vi "Logger Table.vi"() -> ()   [LabVIEW 2019]
uses:
  <vilib>/Analysis/NI_AALBase.lvlib
panel:
  out "x/y 3":dbl
  out "x/y 2":dbl
  out "x/y":dbl
  in  "Weighting (Sample)":enum16{"Sample", "Population"}(ring)
  out "standard deviation 3":dbl format="%.3f"
  out "variance 3":dbl format="%.10f"
  out "Waveform Graph":dbl[](graph)
  out "variance 2":dbl format="%.10f"
  out "variance":dbl format="%.10f"
  in  "samples":i32=100000
  out "standard deviation 2":dbl format="%.3f"
  out "standard deviation":dbl format="%.3f"
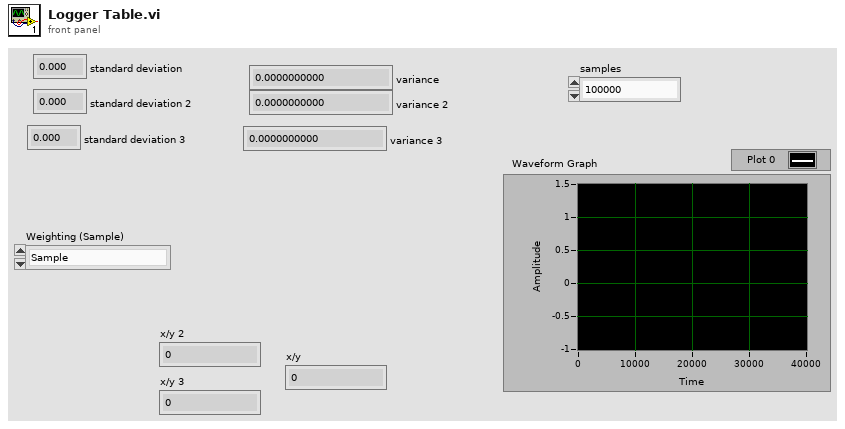
[diagram p1: front panel]
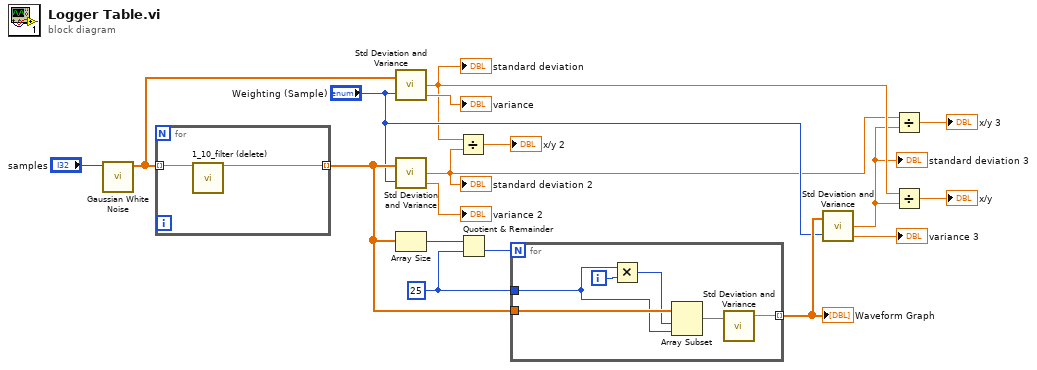
[diagram p0: block diagram]
diagram:
  w11 = 25 ("length")
  n1 = call <vilib>:"Gaussian White Noise.vi"("samples"="samples") -> ("Gaussian noise pattern"=w16:dbl[])  [unwired: 9 in, 1 out]
  n2 = for {
    tunnel: w16 -> [w18] mode=indexing
    tunnel: [w19] -> w13 mode=indexing
    n3 = call "1_10_filter (delete).vi"("input"=w18) -> ("output"=w19:dbl)  [unwired: 14 in]
  }
  n4 = call <vilib>:"Std Deviation and Variance.vi"("X"=w16, "Weighting (Sample)"="Weighting (Sample)") -> ("standard deviation"=w4:dbl, "variance"=→"variance":dbl)  [unwired: 1 out]
  "standard deviation" <- w4
  n5 = call <vilib>:"Std Deviation and Variance.vi"("X"=w13, "Weighting (Sample)"="Weighting (Sample)") -> ("standard deviation"=w2:dbl, "variance"=→"variance 2":dbl)  [unwired: 1 out]
  "standard deviation 2" <- w2
  n6 = Array Size(array=w13) -> (size(s)=w12:i32)
  n7 = Divide(x=w4, y=w2) -> (x/y=→"x/y 2":dbl)
  n8 = Quotient & Remainder(x=w12, y=w11) -> (floor(x/y)=w10:i32)  [unwired: 1 out]
  n9 = for {
    N: w10 -> [_]
    tunnel: w13 -> [w25]
    tunnel: w11 -> [w21]
    tunnel: [w20] -> w8 mode=indexing
    i -> [w23]
    n10 = Multiply(x=w21, y=w23) -> (x*y=w22:i32)
    n11 = Array Subset(array=w25, index=w22, length=w21) -> (w24:dbl[])
    n12 = call <vilib>:"Std Deviation and Variance.vi"("X"=w24) -> ("mean"=w20:dbl)  [unwired: 1 in, 2 out]
  }
  "Waveform Graph" <- w8
  n13 = call <vilib>:"Std Deviation and Variance.vi"("X"=w8, "Weighting (Sample)"="Weighting (Sample)") -> ("standard deviation"=w1:dbl, "variance"=→"variance 3":dbl)  [unwired: 1 out]
  "standard deviation 3" <- w1
  n14 = Divide(x=w2, y=w1) -> (x/y=→"x/y 3":dbl)
  n15 = Divide(x=w4, y=w1) -> (x/y=→"x/y":dbl)
